vi "Heater Device (Read).vi"(6 "ISOBUS address":T5=-1 caption="ISOBUS address (-1)", 8 "error in":errorcluster, 11 "Mercury Reference In":T6) -> (0 "error out":errorcluster, 2 "Device Details":T2, 3 "Mercury Reference Out":T6, 4 "Valid?":T1)   [LabVIEW 2014, in "Mercury iXX.lvlib" / "Heater.lvlib"]
doc: "Read the current device configuration for the selected heater device."
uses:
  Heater.lvlib
  Controls/Mercury Reference.ctl
  Controls/Comms Transport Layer.ctl
  Private/Controls/Query Dynamic Reference.ctl
  Controls/ISOBus Address.ctl
  Controls/Heater Device (Read).ctl
  Controls/Manufacturing Data.ctl
  Controls/Heater Signals Cluster.ctl
  Controls/Is Valid LED.ctl
  Private/Controls/Command Verbs.ctl
  Mercury iXX.lvlib
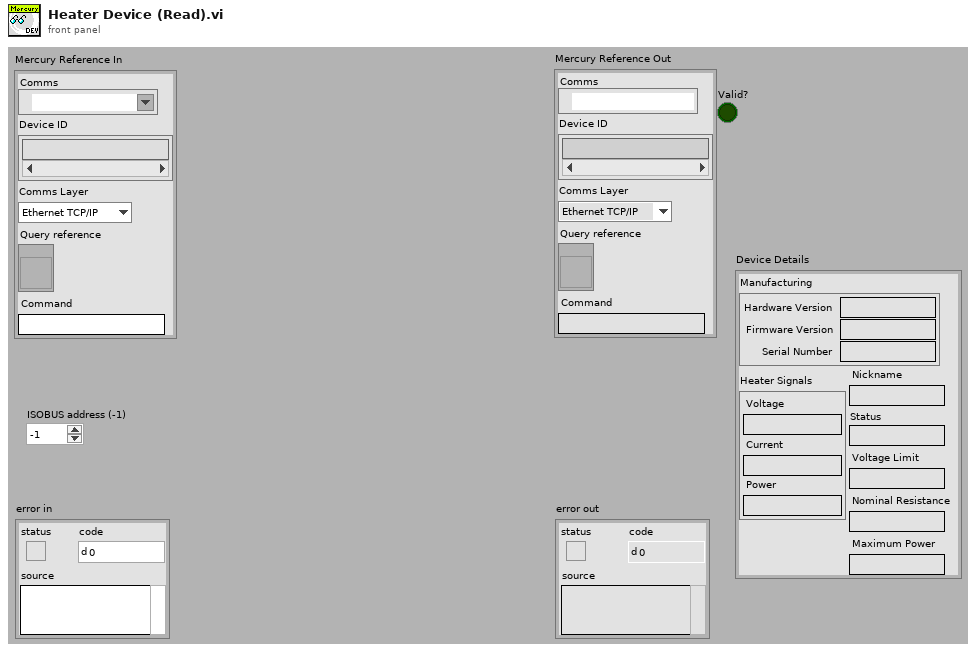
[diagram p1: front panel]
types:
  T1 = typedef "Mercury iXX.lvlib/Is Valid LED.ctl" = bool
  T2 = typedef "Mercury iXX.lvlib/Heater.lvlib/Heater Device (Read).ctl" = cluster{"Manufacturing":T3, "Nickname":string, "Voltage Limit":string, "Nominal Resistance":string, "Maximum Power":string, "Heater Signals":T4, "Status":string}
  T3 = typedef "Mercury iXX.lvlib/Manufacturing Data.ctl" = cluster{"Hardware Version":string, "Firmware Version":string, "Serial Number":string}
  T4 = typedef "Mercury iXX.lvlib/Heater.lvlib/Heater Signals Cluster.ctl" = cluster{"Voltage":string, "Current":string, "Power":string}
  T5 = typedef "Mercury iXX.lvlib/ISOBus Address.ctl" = i32
  T6 = typedef "Mercury iXX.lvlib/Mercury Reference.ctl" = cluster{"Comms":refnum<visa-resource-name>, "Device ID":string[], "Comms Layer":T7, "Command":string, "Query reference":T8}
  T7 = typedef "Mercury iXX.lvlib/Comms Transport Layer.ctl" = enum16{"Ethernet TCP/IP", "USB", "ISOBus - RS-232", "GPIB"}
  T8 = typedef "Mercury iXX.lvlib/Query Dynamic Reference.ctl" = refnum<vi>
  T9 = typedef "Mercury iXX.lvlib/Command Verbs.ctl" = string
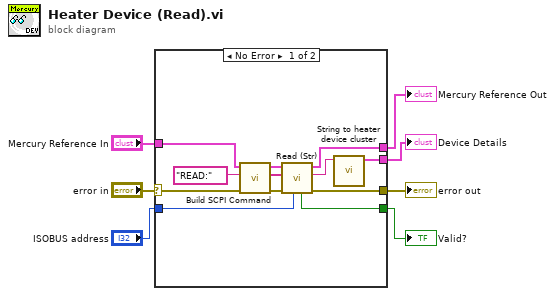
[diagram p0: block diagram]
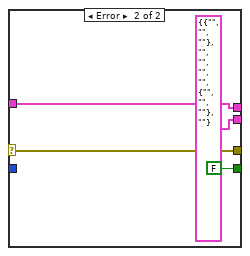
[diagram p2: hidden frame]
diagram:
  n1 = case shown="No Error" "error in" {
    selector: "error in" -> [w8 w23]
    tunnel: [w19 T2 {"Manufacturing"={"Hardware Version"="", "Firmware Version"="", "Serial Number"=""}, "Nickname"="", "Voltage Limit"="", "Nominal Resistance"="", "Maximum Power"="", "Heater Signals"={"Voltage"="", "Current"="", "Power"=""}, "Status"=""} ("Heater Device Settings")] -> w7
    tunnel: [w14 w22] -> w6
    tunnel: [w12 w23] -> w5
    tunnel: [w11 T1 FALSE ("Valid?")] -> w4
    tunnel: "ISOBUS address" -> [w10 _]
    tunnel: "Mercury Reference In" -> [w9 w22]
    frame No Error {
      n2 = call "Build SCPI Command.vi"("error in"=w8, "Verb"=T9 "READ:", "Mercury Reference In"=w9) -> ("error out"=w18:errorcluster, "SCPI Message(s)"=w15:string[], "Mercury Reference Out"=w16:T6)  [unwired: 1 in, 5 out]
      n3 = call "Read (Str).vi"("ISOBUS address"=w10, "error in"=w18, "SCPI Message(s)"=w15, "Mercury Reference In"=w16) -> ("error out"=w12:errorcluster, "Response"=w13:string, "Mercury Reference Out"=w14:T6, "Valid?"=w11:T1)  [unwired: 4 out]
      n4 = call "String to heater device cluster.vi"("HTR Device Details"=w13) -> ("Heater Device Settings"=w19:T2)  [unwired: 10 out]
    }
    frame Error {
    }
  }
  "Mercury Reference Out" <- w6
  "error out" <- w5
  "Device Details" <- w7
  "Valid?" <- w4
